vi "FABR-Update Analysis.vi"(0 "Analysis in":T2, 7 "update":T1[](array[typedef]), 11 "error in (no error)":errorcluster) -> (3 "progress":dbl, 4 "Analysis out":T2, 8 "finished":bool, 15 "error out":errorcluster)   [LabVIEW 2020]
uses:
  Typedefs/FABR-Analysis State.ctl
  Threshold Estimation VIs/ABR3-Threshold Estimation Result.ctl
  Typedefs/FABR-Stimulus Condition.ctl
panel:
  # "Freq X Level X Time"
  # "Freq X Level X Time"
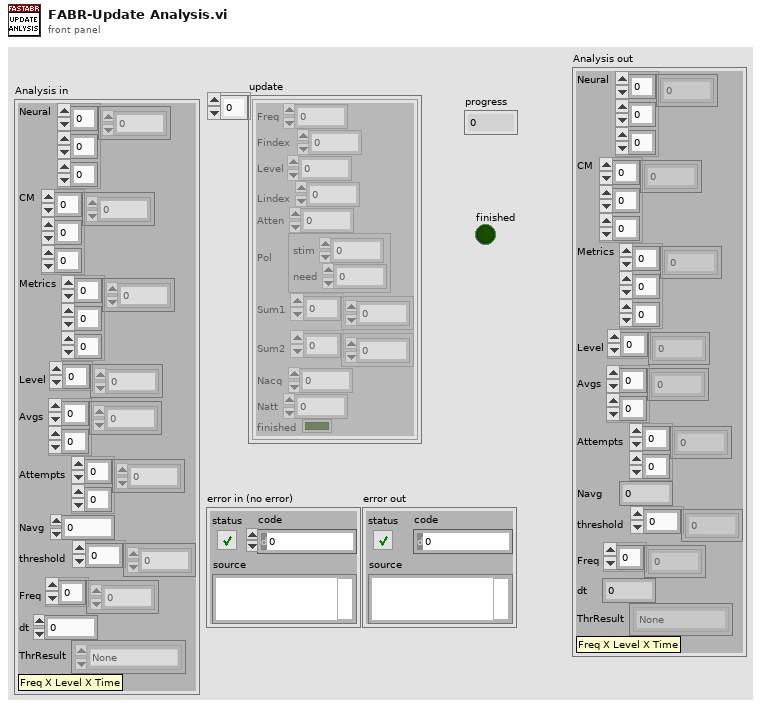
[diagram p1: front panel]
types:
  T1 = typedef "FABR-Stimulus Condition.ctl" = cluster{"Freq":dbl, "Findex":i32, "Level":dbl, "Lindex":i32, "Atten":dbl, "Pol":cluster{"stim":i32, "need":i32}, "Sum1":dbl[], "Sum2":dbl[], "Nacq":i32, "Natt":i32, "finished":bool}
  T2 = typedef "FABR-Analysis State.ctl" = cluster{"Neural":dbl[][][], "CM":dbl[][][], "Metrics":dbl[][][], "Level":dbl[], "Avgs":i32[][], "Attempts":i32[][], "Navg":i32, "threshold":dbl[], "Freq":dbl[], "dt":dbl, "ThrResult":T3[]}
  T3 = typedef "ABR3-Threshold Estimation Result.ctl" = enum16{"None", "Power", "Sigmoid", "Power (noisy)", "Suprathreshold", "Invalid"}
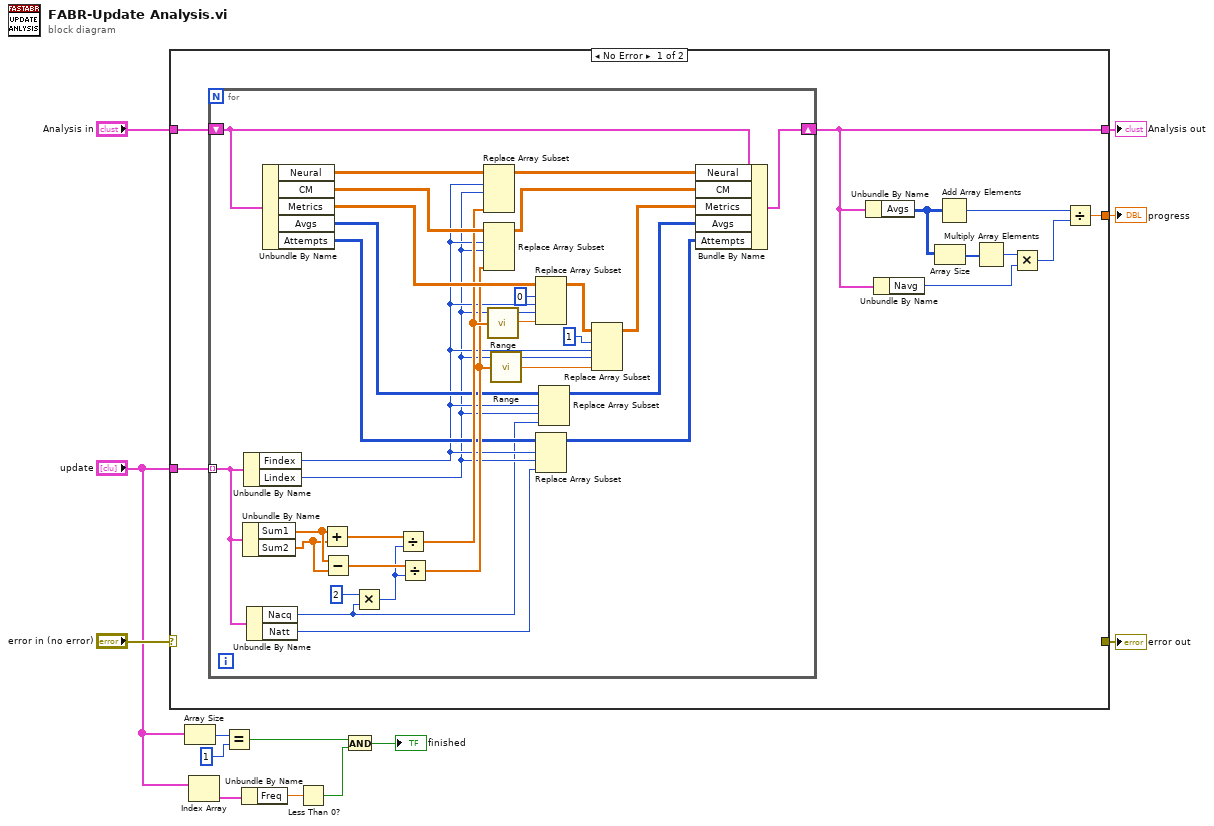
[diagram p0: block diagram]
diagram:
  n1 = case shown="No Error" "error in (no error)" {
    selector: "error in (no error)" -> [_ w55]
    tunnel: "update" -> [w23 _]
    tunnel: "Analysis in" -> [w22 w54]
    tunnel: [w18 w54] -> w12
    tunnel: [_ w55] -> w10
    tunnel: [w14 _] -> w1
    frame No Error {
      n2 = for {
        tunnel: w23 -> [w48] mode=indexing
        shift-right: [w43] -> w18
        shift-left: w22 -> [w46]
        n3 = Unbundle By Name(w48) -> ("Sum1"=w52:dbl[], "Sum2"=w51:dbl[])
        n4 = Unbundle By Name(w48) -> ("Findex"=w30:i32, "Lindex"=w29:i32)
        n5 = Unbundle By Name(w48) -> ("Nacq"=w25:i32, "Natt"=w28:i32)
        n6 = Unbundle By Name(w46) -> ("Neural"=w49:dbl[][][], "CM"=w47:dbl[][][], "Metrics"=w42:dbl[][][], "Avgs"=w33:i32[][], "Attempts"=w31:i32[][])
        n7 = Add(x=w52, y=w51) -> (x+y=w53:dbl[])
        n8 = Subtract(x=w52, y=w51) -> (x-y=w50:dbl[])
        n9 = Multiply(x=2, y=w25) -> (x*y=w26:i32)
        n10 = Divide(x=w53, y=w26) -> (x/y=w41:dbl[])
        n11 = Divide(x=w50, y=w26) -> (x/y=w38:dbl[])
        n12 = Replace Array Subset(array=w49, new element=w41, index (dim 0)=w30, index (dim 1)=w29) -> (w45:dbl[][][])  [unwired: 1 in]
        n13 = Replace Array Subset(array=w47, new element=w38, index (dim 0)=w30, index (dim 1)=w29) -> (w44:dbl[][][])  [unwired: 1 in]
        n14 = call "Range.vi"("Array"=w41) -> ("Range"=w39:dbl)
        n15 = call "Range.vi"("Array"=w38) -> ("Range"=w35:dbl)
        n16 = Replace Array Subset(array=w42, new element=w39, index (dim 0)=0 ("disabled index (page)"), index (dim 1)=w30, index (dim 2)=w29) -> (w37:dbl[][][])
        n17 = Replace Array Subset(array=w31, new element=w28, index (row)=w30, index (col)=w29) -> (w27:i32[][])
        n18 = Replace Array Subset(array=w33, new element=w25, index (row)=w30, index (col)=w29) -> (w32:i32[][])
        n19 = Replace Array Subset(array=w37, new element=w35, index (dim 0)=1 ("disabled index (page)"), index (dim 1)=w30, index (dim 2)=w29) -> (w36:dbl[][][])
        n20 = Bundle By Name(cluster=w46, "Neural"=w45, "CM"=w44, "Metrics"=w36, "Avgs"=w32, "Attempts"=w27) -> (w43:T2)
      }
      n21 = Unbundle By Name(w18) -> ("Avgs"=w21:i32[][])
      n22 = Unbundle By Name(w18) -> ("Navg"=w17:i32)
      n23 = Array Size(array=w21) -> (size(s)=w20:i32[])
      n24 = Add Array Elements(numeric array=w21) -> (sum=w16:i32)
      n25 = Multiply Array Elements(1:w20) -> (0:w19:i32)
      n26 = Multiply(x=w19, y=w17) -> (x*y=w15:i32)
      n27 = Divide(x=w16, y=w15) -> (x/y=w14:dbl)
    }
    frame Error {
    }
  }
  "Analysis out" <- w12
  "error out" <- w10
  "progress" <- w1
  n28 = Array Size(array="update") -> (size(s)=w9:i32)
  n29 = Index Array(array="update") -> (element=w6:T1)  [unwired: 1 in]
  n30 = Equal?(x=w9, y=1) -> (x = y?=w3:bool)
  n31 = Unbundle By Name(w6) -> ("Freq"=w5:dbl)
  n32 = Less Than 0?(x=w5) -> (x < 0?=w4:bool)
  n33 = And(x=w3, y=w4) -> (x .and. y?=→"finished":bool)
